vi "TIO Stream Open_Ser.vi"(8 "error in (no error)":errorcluster, 9 "Port Timeout":u32=500, 10 "Baud Rate":u32=115200, 11 "Nom de ressource VISA":refnum<visa-resource-name>) -> (0 "error out":errorcluster, 1 "Connected":bool=TRUE, 3 "Nom de ressource VISA Out":refnum<visa-resource-name>)   [LabVIEW 2010]
uses:
  <vilib>/Instr/_visa.llb/VISA Configure Serial Port (Instr).vi
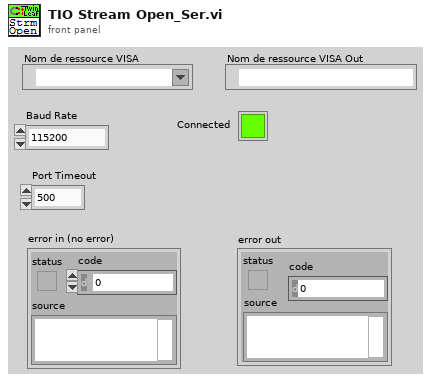
[diagram p1: front panel]
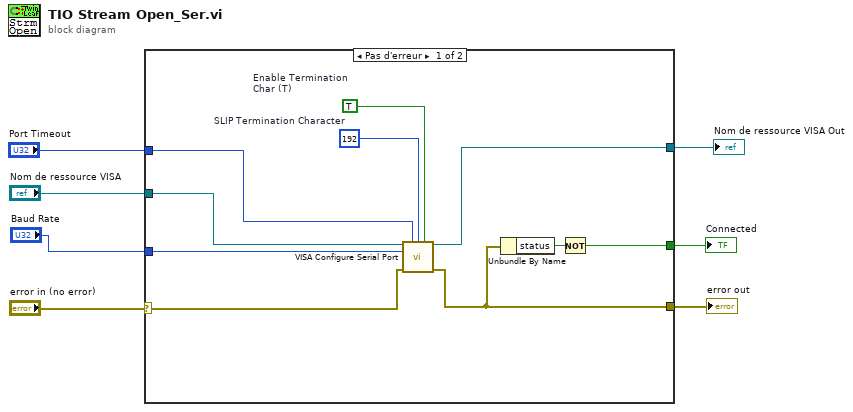
[diagram p0: block diagram]
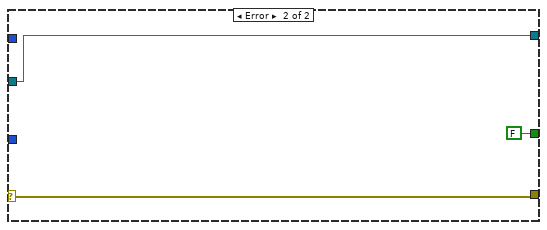
[diagram p2: hidden frame]
diagram:
  n1 = case shown="Pas d'erreur" "error in (no error)" {
    selector: "error in (no error)" -> [w8 w19]
    tunnel: [w17 w19] -> w7
    tunnel: [w15 FALSE] -> w6
    tunnel: "Nom de ressource VISA" -> [w12 w18]
    tunnel: [w11 w18] -> w4
    tunnel: "Port Timeout" -> [w10 _]
    tunnel: "Baud Rate" -> [w9 _]
    frame No Error {
      w13 = TRUE  # Enable Termination Char (T)
      w14 = u8 192  # SLIP Termination Character
      n2 = call-poly "VISA Configure Serial Port"("VISA resource name"=w12, "timeout (10sec)"=w10, "termination char\n(0xA = '\\n' = LF)"=w14, "Enable Termination\nChar (T)"=w13, "baud rate (9600)"=w9, "error in (no error)"=w8) -> ("VISA resource name out"=w11:refnum<visa-resource-name>, "error out"=w17:errorcluster)  [unwired: 8 in]
      n3 = Unbundle By Name(w17) -> ("status"=w16:bool)
      n4 = Not(x=w16) -> (.not. x?=w15:bool)
    }
    frame Error {
    }
  }
  "error out" <- w7
  "Connected" <- w6
  "Nom de ressource VISA Out" <- w4
